vi "Hc2SequenceRunner.vi"() -> ()   [LabVIEW 2019]
uses:
  DeltaRamp_globals.vi
  B_Globals.vi
  Global 2.vi
panel:
  out "Numeric":i32
  in  "Settle [s]":dbl
  in  "Base Name":string
  in  "Start":bool
  in  "Directory":path
  in  "T_high":dbl
  in  "T_low":dbl
  in  "T_rate":dbl
  in  "B _rate":dbl
  in  "Set Fields":dbl[](array[numeric])
  out "Action":string="Waiting for go"
  out "Output File":path
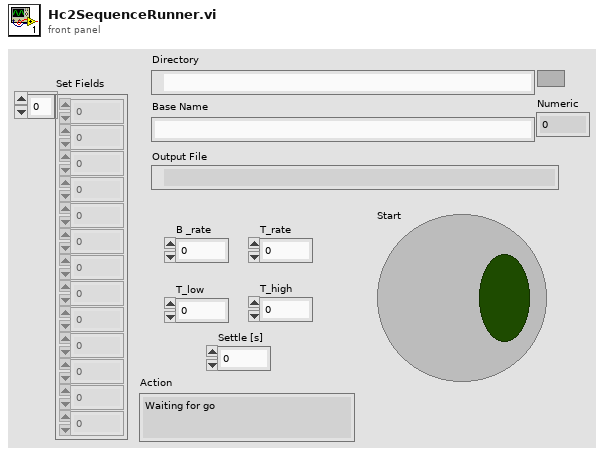
[diagram p1: front panel]
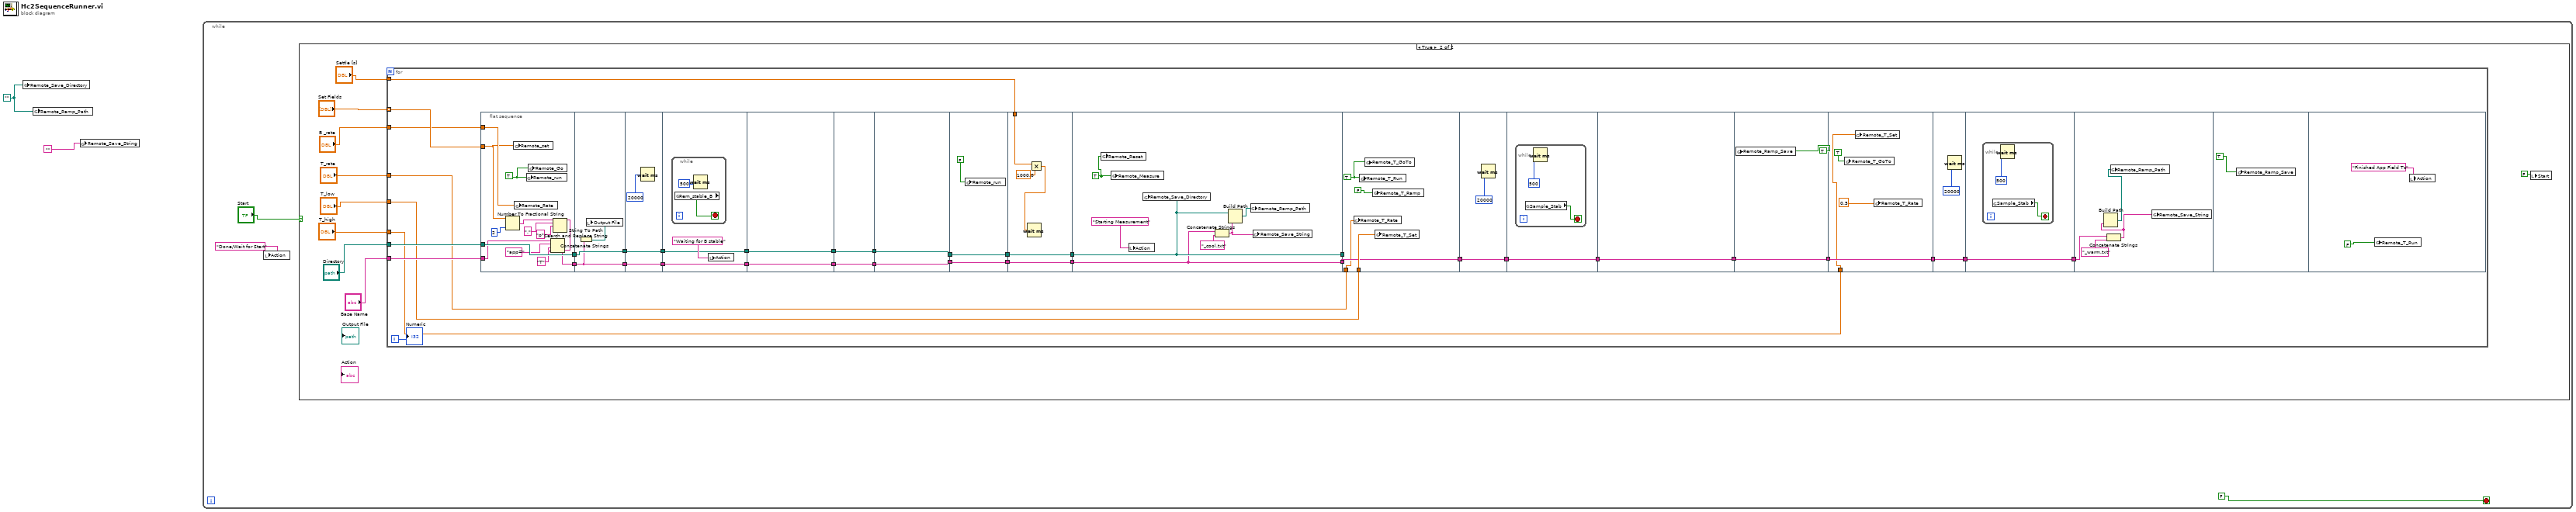
[diagram p0: block diagram]
diagram:
  w2 = path ""
  n1 = global write "DeltaRamp_globals.vi" "Remote_Save_Directory"(w2) -> ()
  n2 = global write "DeltaRamp_globals.vi" "Remote_Ramp_Path"(w2) -> ()
  n3 = global write "DeltaRamp_globals.vi" "Remote_Save_String"("") -> ()
  n4 = while {
    stop <- FALSE stop-if-true
    n5 = local write "Action"("Done/Wait for Start") -> ()
    n6 = case shown="True" "Start" {
      frame False {
      }
      frame True {
        n7 = for {
          tunnel: "Set Fields" -> [w23] mode=indexing
          tunnel: "B _rate" -> [w22]
          tunnel: "Directory" -> [w21]
          tunnel: "Base Name" -> [w20]
          tunnel: "Settle [s]" -> [w19]
          tunnel: "T_low" -> [w18]
          tunnel: "T_rate" -> [w17]
          tunnel: "T_high" -> [w16]
          i -> [w15]
          n8 = flat-sequence {
            tunnel: w23 -> [w59]
            tunnel: w22 -> [w63]
            tunnel: w20 -> [w61]
            tunnel: [w53] -> w51
            tunnel: [w62] -> w50
            tunnel: w21 -> [w62]
            tunnel: [w66] -> w49
            tunnel: w51 -> [w66]
            tunnel: w50 -> [w67]
            tunnel: [w67] -> w48
            tunnel: w49 -> [w70]
            tunnel: [w70] -> w47
            tunnel: w48 -> [w69]
            tunnel: [w69] -> w46
            tunnel: [w72] -> w45
            tunnel: w47 -> [w72]
            tunnel: [w71] -> w44
            tunnel: w46 -> [w71]
            tunnel: [w77] -> w43
            tunnel: w45 -> [w77]
            tunnel: [w76] -> w42
            tunnel: w44 -> [w76]
            tunnel: [w79] -> w41
            tunnel: w43 -> [w79]
            tunnel: [w78] -> w40
            tunnel: w42 -> [w78]
            tunnel: [w81] -> w39
            tunnel: w41 -> [w81]
            tunnel: [w80] -> w38
            tunnel: w40 -> [w80]
            tunnel: w39 -> [w82]
            tunnel: w38 -> [w83]
            tunnel: [w83] -> w37
            tunnel: [w82] -> w36
            tunnel: w19 -> [w88]
            tunnel: [w86] -> w35
            tunnel: w37 -> [w86]
            tunnel: [w85] -> w34
            tunnel: w36 -> [w85]
            tunnel: [w94] -> w33
            tunnel: w35 -> [w94]
            tunnel: [w92] -> w32
            tunnel: w34 -> [w92]
            tunnel: w18 -> [w100]
            tunnel: w33 -> [_]
            tunnel: w32 -> [w98]
            tunnel: [w98] -> w31
            tunnel: w17 -> [w97]
            tunnel: [w102] -> w30
            tunnel: w31 -> [w102]
            tunnel: w30 -> [w104]
            tunnel: [w104] -> w29
            tunnel: w29 -> [w107]
            tunnel: [w107] -> w28
            tunnel: w28 -> [w109]
            tunnel: [w109] -> w27
            tunnel: w27 -> [w111]
            tunnel: [w111] -> w26
            tunnel: w16 -> [w110]
            tunnel: [w114] -> w25
            tunnel: w26 -> [w114]
            tunnel: w25 -> [w116]
            tunnel: [w116] -> w24
            tunnel: w24 -> [w121]
            frame #0 {
              w64 = TRUE
              n9 = Number To Fractional String(number=w59, precision (6)=2) -> (F-format string=w58:string)  [unwired: 2 in]
              n10 = global write "B_Globals.vi" "Remote_set"(w59) -> ()
              n11 = global write "B_Globals.vi" "Remote_Rate"(w63) -> ()
              n12 = global write "B_Globals.vi" "Remote_run"(w64) -> ()
              n13 = global write "B_Globals.vi" "Remote_Go"(w64) -> ()
              n14 = Search and Replace String(input string=w58, search string=".", replace string="p") -> (result string=w55:string)  [unwired: 5 in, 3 out]
              n15 = Concatenate Strings(w61, "app=", w55, "T") -> (w53:string)
            }
            frame #1 {
              n16 = String To Path(string=w66) -> (path=w65:path)
              n17 = local write "Output File"(w65) -> ()
            }
            frame #2 {
              n18 = Wait (ms)(milliseconds to wait=20000) -> ()  [unwired: 1 out]
            }
            frame #3 {
              n19 = while {
                stop <- w74 stop-if-true
                n20 = global read "B_Globals.vi" "Rem_stable_B"() -> (w74:bool)
                n21 = Wait (ms)(milliseconds to wait=500) -> ()  [unwired: 1 out]
              }
              n22 = local write "Action"("Waiting for B stable") -> ()
            }
            frame #4 {
            }
            frame #5 {
            }
            frame #6 {
            }
            frame #7 {
              n23 = global write "B_Globals.vi" "Remote_run"(FALSE) -> ()
            }
            frame #8 {
              n24 = Multiply(x=w88, y=1000.0) -> (x*y=w87:dbl)
              n25 = Wait (ms)(milliseconds to wait=w87) -> ()  [unwired: 1 out]
            }
            frame #9 {
              w96 = TRUE
              n26 = global write "DeltaRamp_globals.vi" "Remote_Reset"(w96) -> ()
              n27 = global write "DeltaRamp_globals.vi" "Remote_Measure"(w96) -> ()
              n28 = local write "Action"("Starting Measurement") -> ()
              n29 = global write "DeltaRamp_globals.vi" "Remote_Save_Directory"(w94) -> ()
              n30 = Concatenate Strings(w92, "_cool.txt") -> (w90:string)
              n31 = Build Path(base path=w94, name or relative path=w90) -> (appended path=w91:path)
              n32 = global write "DeltaRamp_globals.vi" "Remote_Ramp_Path"(w91) -> ()
              n33 = global write "DeltaRamp_globals.vi" "Remote_Save_String"(w90) -> ()
            }
            frame #10 {
              w101 = TRUE
              n34 = global write "Global 2.vi" "Remote_T_Rate"(w97) -> ()
              n35 = global write "Global 2.vi" "Remote_T_Run"(w101) -> ()
              n36 = global write "Global 2.vi" "Remote_T_GoTo"(w101) -> ()
              n37 = global write "Global 2.vi" "Remote_T_Ramp"(FALSE) -> ()
              n38 = global write "Global 2.vi" "Remote_T_Set"(w100) -> ()
            }
            frame #11 {
              n39 = Wait (ms)(milliseconds to wait=20000) -> ()  [unwired: 1 out]
            }
            frame #12 {
              n40 = while {
                stop <- w106 stop-if-true
                n41 = global read "Global 2.vi" "Sample_Stab"() -> (w106:bool)
                n42 = Wait (ms)(milliseconds to wait=500) -> ()  [unwired: 1 out]
              }
            }
            frame #13 {
            }
            frame #14 {
              n43 = global write "DeltaRamp_globals.vi" "Remote_Ramp_Save"(TRUE) -> ()
            }
            frame #15 {
              n44 = global write "Global 2.vi" "Remote_T_GoTo"(TRUE) -> ()
              n45 = global write "Global 2.vi" "Remote_T_Set"(w110) -> ()
              n46 = global write "Global 2.vi" "Remote_T_Rate"(0.5) -> ()
            }
            frame #16 {
              n47 = Wait (ms)(milliseconds to wait=20000) -> ()  [unwired: 1 out]
            }
            frame #17 {
              n48 = while {
                stop <- w118 stop-if-true
                n49 = global read "Global 2.vi" "Sample_Stab"() -> (w118:bool)
                n50 = Wait (ms)(milliseconds to wait=500) -> ()  [unwired: 1 out]
              }
            }
            frame #18 {
              n51 = Concatenate Strings(w121, "_warm.txt") -> (w119:string)
              n52 = Build Path(name or relative path=w119) -> (appended path=w120:path)  [unwired: 1 in]
              n53 = global write "DeltaRamp_globals.vi" "Remote_Ramp_Path"(w120) -> ()
              n54 = global write "DeltaRamp_globals.vi" "Remote_Save_String"(w119) -> ()
            }
            frame #19 {
              n55 = global write "DeltaRamp_globals.vi" "Remote_Ramp_Save"(TRUE) -> ()
            }
            frame #20 {
              n56 = global write "Global 2.vi" "Remote_T_Run"(FALSE) -> ()
              n57 = local write "Action"("Finished App Field Tc") -> ()
            }
          }
          "Numeric" <- w15
        }
        n58 = local write "Start"(FALSE) -> ()
      }
    }
  }
